vi "IsErrorCluster.vi"(8 "error in (no error)":errorcluster, 11 "Variant":variant) -> (0 "error out":errorcluster, 2 "Is Error Cluster":bool)   [LabVIEW 2017, in "LVUnitTestBuilder.lvclass"]
doc: "Returns true if <B>Variant</B> is an Error Cluster."
uses:
  LVUnitTestBuilder.lvclass
  <vilib>/Utility/Data Type/NI_Data Type.lvlib
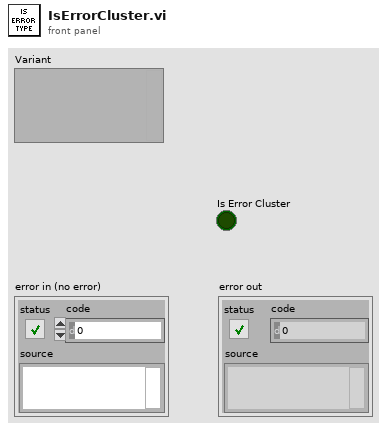
[diagram p1: front panel]
types:
  T1 = typedef "NI_Data Type.lvlib/Data Type.ctl" = enum8{"Invalid Type", "Void", "I8", "I16", "I32", "I64", "U8", "U16", "U32", "U64", "Single Float", "Double Float", "Extended Float", "Single Complex", "Double Complex", "Extended Complex", "Enum U8", "Enum U16", "Enum U32", "Enum U64", "Single Float With Unit", "Double Float With Unit", "Extended Float With Unit", "Single Complex with Unit", "Double Complex with Unit", "Extended Complex with Unit", "Boolean", "String", "Path", "Picture", "Tag", "Array", "Cluster", "Variant", "LV Variant", "Waveform", "Timestamp", "Digital Waveform", "Digital Data", "ExpressData", "Refnum", "External Data", "VI", "Poly VI", "LabVIEW Class Instance", "Fixed Point"}
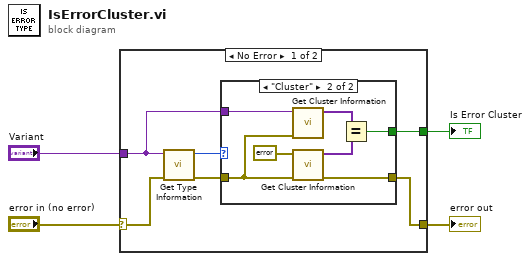
[diagram p0: block diagram]
diagram:
  n1 = case shown="No Error" "error in (no error)" {
    selector: "error in (no error)" -> [w6 w19]
    tunnel: "Variant" -> [w9 _]
    tunnel: [w8 _] -> w3
    tunnel: [w5 w19] -> w1
    frame No Error {
      n2 = call <vilib>:"Get Type Information.vi"("error in (no error)"=w6, "Variant"=w9) -> ("error out"=w7:errorcluster, "Type"=w10:T1)  [unwired: 5 in, 3 out]
      n3 = case shown="\"Cluster\"" w10 {
        tunnel: w9 -> [_ w18]
        tunnel: [_ w14] -> w8
        tunnel: w7 -> [w11 w13]
        tunnel: [w11 w12] -> w5
        frame Default {
        }
        frame "Cluster" {
          n4 = call <vilib>:"Get Cluster Information.vi"("error in (no error)"=w13, "Variant"=w18) -> ("Cluster Elements"=w17:variant[])  [unwired: 8 in, 1 out]
          n5 = call <vilib>:"Get Cluster Information.vi"("error in (no error)"=w13, "Variant"=errorcluster {"status"=FALSE, "code"=0, "source"=""} ("error in (no error)")) -> ("error out"=w12:errorcluster, "Cluster Elements"=w16:variant[])  [unwired: 8 in]
          n6 = Equal?(x=w17, y=w16) -> (x = y?=w14:bool)
        }
      }
    }
    frame Error {
    }
  }
  "Is Error Cluster" <- w3
  "error out" <- w1
